vi "Fibonacci.vi"(10 "n":u8) -> (2 "Fib(n)":u8)   [LabVIEW 2015]
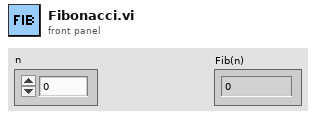
[diagram p1: front panel]
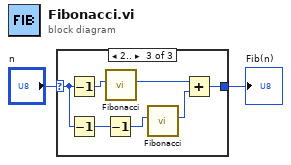
[diagram p0: block diagram]
diagram:
  n1 = case shown="2.." "n" {
    selector: "n" -> [w3 w4 w11]
    tunnel: [w3 w4 w5] -> w1
    frame 0, Default {
    }
    frame 1 {
    }
    frame 2.. {
      n2 = Decrement(x=w11) -> (x-1=w9:u8)
      n3 = Decrement(x=w11) -> (x-1=w10:u8)
      n4 = Decrement(x=w10) -> (x-1=w8:u8)
      n5 = call "Fibonacci.vi"("n"=w9) -> ("Fib(n)"=w7:u8)  [unwired: 10 in]
      n6 = call "Fibonacci.vi"("n"=w8) -> ("Fib(n)"=w6:u8)  [unwired: 10 in]
      n7 = Add(x=w7, y=w6) -> (x+y=w5:u8)
    }
  }
  "Fib(n)" <- w1
